vi "UART List.vi"(8 "error in (no error)":errorcluster) -> (0 "error out":errorcluster, 1 "Ports #":i32, 2 "Serial Ports":string[](array[string]), 3 "Success?":bool)   [LabVIEW 2013]
uses:
  filter wheel/Libraries/uart_library.dll
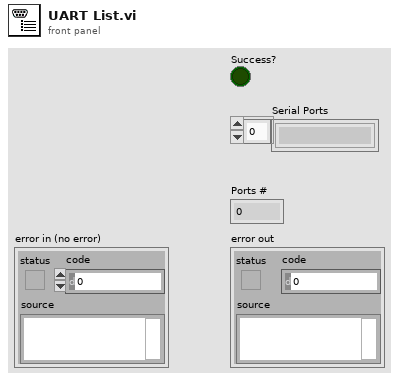
[diagram p1: front panel]
types:
  T1 = cluster{"offset past number":i32, "Name":string}[]
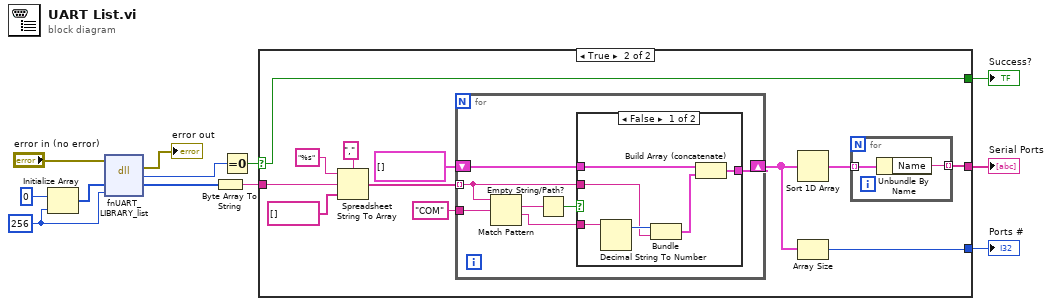
[diagram p0: block diagram]
diagram:
  w3 = 256 ("Var")
  n1 = Initialize Array(u8 0 ("element"), w3) -> (w4:u8[])
  n2 = dll-call lib="E:/users/tba/work_project/FW102/trunk/LabVIEW/Libraries/uart_library.dll" fn="fnUART_LIBRARY_list"(error in="error in (no error)", "nPort"=w4, "Var"=w3) -> (error out=→"error out":errorcluster, "return type"=w10:i32, "nPort"=w2:u8[])  [unwired: 3 in, 1 out]
  n3 = Byte Array To String(unsigned byte array=w2) -> (string=w1:string)
  n4 = Equal To 0?(x=w10) -> (x = 0?=w9:bool)
  n5 = case shown="True" w9 {
    selector: w9 -> [w13 w19]
    tunnel: [_ w14] -> w12
    tunnel: [_ w20] -> w11
    tunnel: [w13 w19] -> w8
    tunnel: w1 -> [_ w18]
    frame False {
    }
    frame True {
      n6 = Spreadsheet String To Array(delimiter (Tab)=",", format string="%s", spreadsheet string=w18, array type (2D Dbl)=string[] []) -> (array=w22:string[])
      n7 = for {
        tunnel: w22 -> [w31] mode=indexing
        shift-right: [w34] -> w21
        shift-left: cluster{"ID":i32, "Name":string}[] [] -> [w33]
        tunnel: "COM" ("regular expression") -> [w30]
        n8 = Match Pattern(string=w31, regular expression=w30) -> (match substring=w29:string, after substring=w28:string)  [unwired: 1 in, 2 out]
        n9 = Empty String/Path?(string/path=w29) -> (empty?=w32:bool)
        n10 = case shown="False" w32 {
          tunnel: w31 -> [w36 _]
          tunnel: [w40 w41] -> w34
          tunnel: w33 -> [w39 w41]
          tunnel: w28 -> [w38 _]
          frame False {
            n11 = Decimal String To Number(string=w38) -> (offset past number=w37:i32)  [unwired: 2 in, 1 out]
            n12 = Bundle("offset past number"=w37, w36) -> (w35:cluster{"offset past number":i32, string})  [unwired: 1 in]
            n13 = Build Array (concatenate)(w39, w35) -> (w40:T1)
          }
          frame True {
          }
        }
      }
      n14 = Sort 1D Array(array=w21) -> (sorted array=w15:cluster{"ID":i32, "Name":string}[])
      n15 = Array Size(array=w21) -> (size(s)=w20:i32)
      n16 = for {
        tunnel: w15 -> [w27] mode=indexing
        tunnel: [w26] -> w14 mode=indexing
        n17 = Unbundle By Name(w27) -> ("Name"=w26:string)
      }
    }
  }
  "Serial Ports" <- w12
  "Ports #" <- w11
  "Success?" <- w8
